vi "Position measurement.vi"(0 "Image":T1, 1 "Trap positions":T2, 2 "ROIs":T1[](array[typedef]), 3 "Follow traps?":bool, 4 "Acquired Buffer Number":u32, 5 "ROI size":dbl=20.0) -> (6 "Position data out":T3)   [LabVIEW 8.6]
uses:
  <vilib>/vision/NI_Vision_Development_Module.lvlib
  Trap cluster.ctl
  <vilib>/vision/Image Controls.llb/IMAQ Image.ctl
panel:
  in  "Display ROI nr":i32
  out "Image 2":T1(plugin-control)
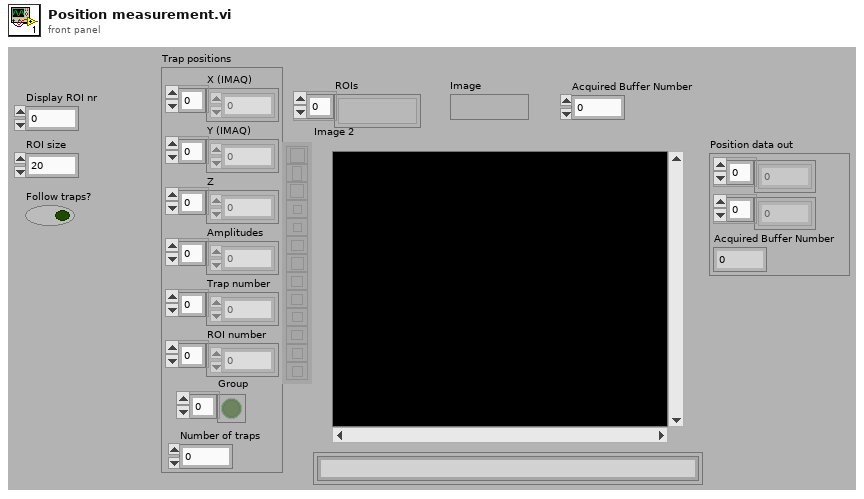
[diagram p1: front panel]
types:
  T1 = typedef "IMAQ Image.ctl" = refnum<image>
  T2 = typedef "Trap cluster.ctl" = cluster{"X (IMAQ)":dbl[], "Y (IMAQ)":dbl[], "Z":dbl[], "Amplitudes":dbl[], "Trap number":i32[], "ROI number":i32[], "Number of traps":i32, "Group":bool[]}
  T3 = cluster{dbl[], dbl[], "Acquired Buffer Number":u32}
  T4 = cluster{"X (IMAQ)":dbl[], "Y (IMAQ)":dbl[], "Acquired Buffer Number":u32}
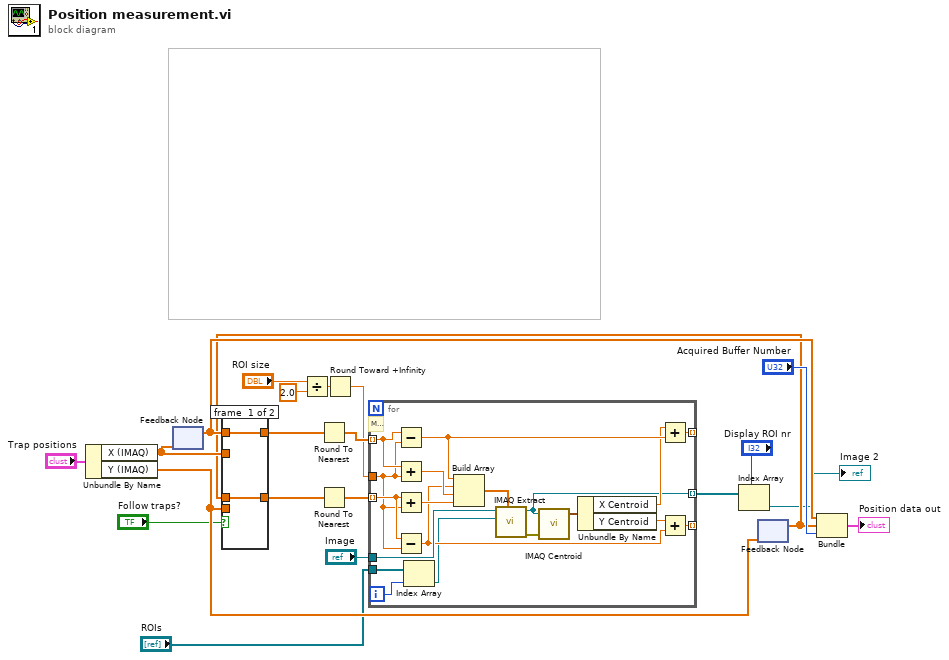
[diagram p0: block diagram]
diagram:
  # "Missing object. The object \"Number of Workers\" does not exist in the previous version."
  n1 = Unbundle By Name("Trap positions") -> ("X (IMAQ)"=w9:dbl[], "Y (IMAQ)"=w6:dbl[])
  n2 = feedback #1(w9) -> (w10:dbl[])
  n3 = Divide(x="ROI size", y=2.0) -> (x/y=w18:dbl)
  n4 = Round Toward +Infinity(x=w18) -> (ceil(x): smallest int >= x=w1:dbl)
  n5 = feedback #2(w6) -> (w7:dbl[])
  n6 = case shown="True" "Follow traps?" {
    tunnel: w9 -> [_ w27]
    tunnel: w6 -> [_ w26]
    tunnel: [w25 w27] -> w13
    tunnel: [w24 w26] -> w12
    tunnel: w10 -> [w25 _]
    tunnel: w7 -> [w24 _]
    frame #0 {
    }
    frame #1 {
    }
  }
  n7 = Round To Nearest(number=w13) -> (nearest integer value=w15:dbl[])
  n8 = Round To Nearest(number=w12) -> (nearest integer value=w14:dbl[])
  n9 = for {
    tunnel: w15 -> [w44] mode=indexing
    tunnel: w14 -> [w43] mode=indexing
    tunnel: "Image" -> [w46]
    tunnel: "ROIs" -> [w45]
    tunnel: w1 -> [w42]
    tunnel: [w32] -> w11 mode=indexing
    tunnel: [w31] -> w8 mode=indexing
    tunnel: [w30] -> w16 mode=indexing
    i -> [w28]
    n10 = Subtract(x=w44, y=w42) -> (x-y=w36:dbl)
    n11 = Add(x=w44, y=w42) -> (x+y=w41:dbl)
    n12 = Add(x=w43, y=w42) -> (x+y=w40:dbl)
    n13 = Subtract(x=w43, y=w42) -> (x-y=w33:dbl)
    n14 = Index Array(array=w45, index=w28) -> (element=w29:T1)
    n15 = Build Array(w36, w33, w41, w40) -> (w39:dbl[])
    n16 = call "IMAQ Extract"("Optional Rectangle"=w39, "Image Dst"=w29, "Image Src"=w46) -> ("error out"=w38:errorcluster, "Image Dst Out"=w30:T1)  [unwired: 7 in]
    n17 = call "IMAQ Centroid"("error in (no error)"=w38, "Image"=w30) -> ("Centroid"=w37:cluster{"X Centroid":sgl, "Y Centroid":sgl})  [unwired: 2 in, 1 out]
    n18 = Unbundle By Name(w37) -> ("X Centroid"=w35:sgl, "Y Centroid"=w34:sgl)
    n19 = Add(x=w35, y=w36) -> (x+y=w32:dbl)
    n20 = Add(x=w34, y=w33) -> (x+y=w31:dbl)
  }
  n21 = Index Array(array=w16, index="Display ROI nr") -> (element=→"Image 2":T1)
  n22 = Bundle("X (IMAQ)"=w10, "Y (IMAQ)"=w7, "Acquired Buffer Number"="Acquired Buffer Number") -> (→"Position data out":T4)  [unwired: 1 in]
